vi "get_sp_from_tb.vi"(7 "lc_num":string) -> (0 "nx_spsta":string, 1 "cur_spnum":string, 2 "error":errorcluster caption="error out 4", 3 "fqren":string)   [LabVIEW 2017, in "Lib_code.lvlib"]
uses:
  Lib_code.lvlib
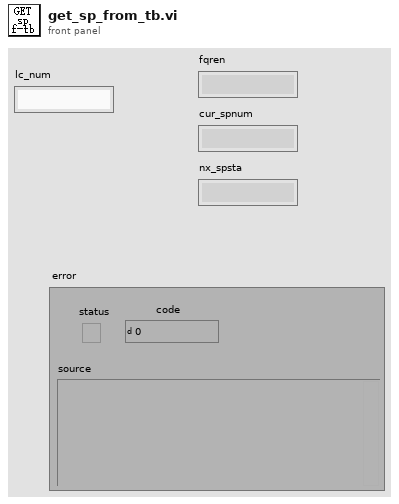
[diagram p1: front panel]
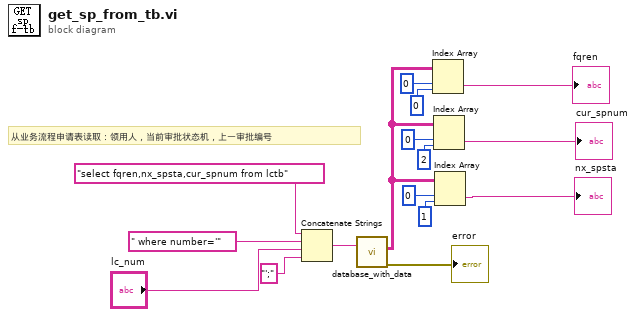
[diagram p0: block diagram]
diagram:
  # "从业务流程申请表读取：领用人，当前审批状态机，上一审批编号"
  n1 = Concatenate Strings("select fqren,nx_spsta,cur_spnum from lctb" ("Command Text"), " where number='" ("Command Text"), "lc_num", "';" ("字符串")) -> (w3:string)
  n2 = call "database_with_data.vi"("input"=w3) -> ("error"=→"error":errorcluster, "Data"=w2:string[][])  [unwired: 9 in]
  n3 = Index Array(array=w2, index (row)=0 ("索引 (行)"), index (col)=0 ("禁用的索引 (列)")) -> (element=→"fqren":string)
  n4 = Index Array(array=w2, index (row)=0 ("索引 (行)"), index (col)=2 ("禁用的索引 (列)")) -> (element=→"cur_spnum":string)
  n5 = Index Array(array=w2, index (row)=0 ("索引 (行)"), index (col)=1 ("禁用的索引 (列)")) -> (element=→"nx_spsta":string)
